vi "Simplified WB Spectrum Sense (Averaged).vi"(7 "Averaging Parameters":T1={"averaging mode"=enum."RMS averaging", "weighting mode"=enum."Linear", "number of averages"=10} {"number of averages" min=1}, 9 "Display Settings":cluster{"display unit":u16, "log/linear":u16}={"display unit"=2, "log/linear"=2} {"log/linear" items=["Linear", "dB", "dBm"]; "display unit" items=["Vrms", "Vpk", "Vrms^2", "Vpk^2", "Vrms/rtHz", "Vpk/rtHz", "Vrms^2/Hz", "Vpk^2/Hz"]}, 10 "Rx Parameters":T2={"IQ Sampling\nRate [S/sec]"=1000000.0, "Acq Duration [sec]"=0.001, "Start Carrier [Hz]"=88000000.0, "Stop Carrier [Hz]"=108000000.0, "Gain [dB]"=25.0, "Active Antenna"="RX2", "Reference Source"="Internal", "Timebase Source"="Internal"} {"Gain [dB]" format="%#_4g"; "Stop Carrier [Hz]" min=50000000.0 max=6000000000.0 step=1000.0 format="%#.15p"; "Start Carrier [Hz]" min=50000000.0 max=6000000000.0 step=1000.0 format="%#.15p"; "Acq Duration [sec]" min=0.0 step=0.001 format="%#.6p"; "IQ Sampling\nRate [S/sec]" format="%#_6p"}, 11 "USRP IP Address":refnum<k15>="192.168.12.4") -> (0 "error out":errorcluster, 2 "FFT Power Spectrum":cluster{"f0":dbl, "df":dbl, "IQ":dbl[]}(graph)={"f0"=87750000.0, "df"=1000.0, "IQ"=array[20500 elements]})   [LabVIEW 2011]
panel:
  in  "stop":bool
  # "Wideband Spectrum (Averaged)"
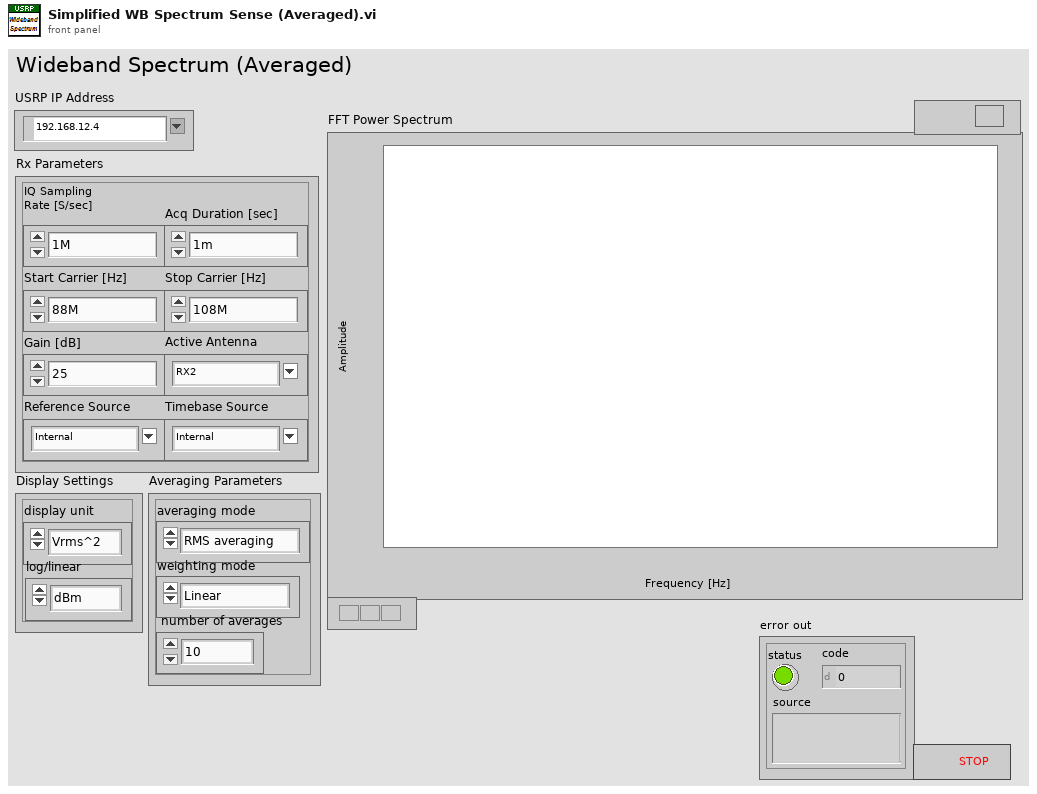
[diagram p1: front panel]
types:
  T1 = cluster{"averaging mode":enum16{"No averaging", "Vector averaging", "RMS averaging", "Peak hold"}, "weighting mode":enum16{"Linear", "Exponential"}, "number of averages":u32}
  T2 = cluster{"IQ Sampling\nRate [S/sec]":dbl, "Acq Duration [sec]":dbl, "Start Carrier [Hz]":dbl, "Stop Carrier [Hz]":dbl, "Gain [dB]":dbl, "Active Antenna":string, "Reference Source":string, "Timebase Source":string}
  T3 = typedef "subFrameParams.ctl" = cluster{"IQ Rate":dbl, "Frames":i32, "Length of Subset":i32, "Start Index of Subset":i32, "Start Carrier [Hz]":dbl, "Stop Carrier [Hz]":dbl, "Acq Duration [sec]":dbl}
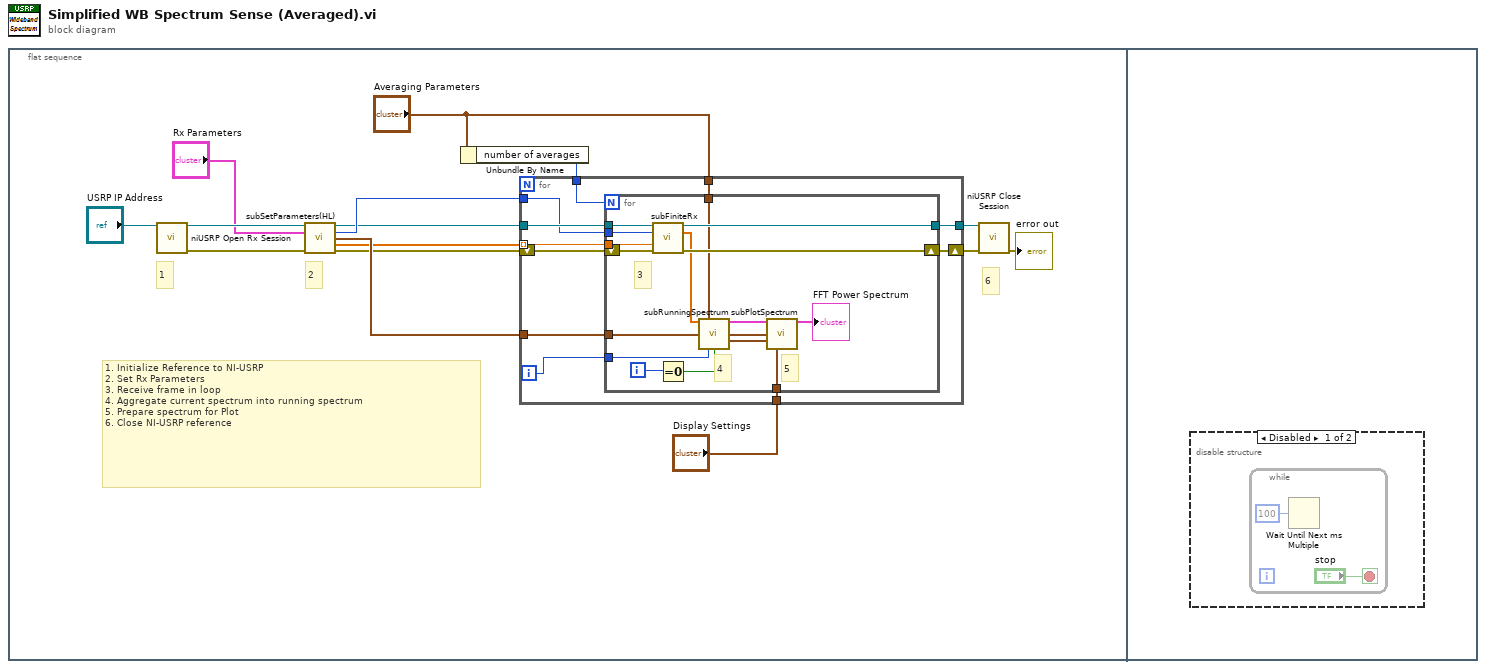
[diagram p0: block diagram]
diagram:
  n1 = flat-sequence {
    frame #0 {
      # "6"
      # "2"
      # "1"
      # "1. Initialize Reference to NI-USRP\n2. Set Rx Parameters\n3. Receive frame in loop\n4. Aggregate current spectrum into running spectrum\n5. Prepare spectrum for Plot\n6. Close NI-USRP reference"
      n2 = call <instrlib>:"niUSRP Open Rx Session.vi"("device names"="USRP IP Address") -> ("session handle out"=w10:refnum<k15>, "error out"=w9:errorcluster)  [unwired: 13 in]
      n3 = call "subSetParameters(HL).vi"("IVI Refnum in"=w10, "Rx Parameters"="Rx Parameters", "error in (no error)"=w9) -> ("IVI Refnum out"=w2:refnum<k15>, "samples per acquisition"=w12:i32, "Frame Parameters"=w7:T3, "test carrier frequencies"=w6:dbl[], "error out"=w1:errorcluster)  [unwired: 8 in]
      n4 = Unbundle By Name("Averaging Parameters") -> ("number of averages"=w4:u32)
      n5 = for {
        tunnel: w2 -> [w26]
        tunnel: w12 -> [w20]
        tunnel: [w25] -> w14
        shift-right: [w19] -> w13
        shift-left: w1 -> [w24]
        tunnel: w7 -> [w23]
        tunnel: w6 -> [w22] mode=indexing
        tunnel: "Display Settings" -> [w21]
        tunnel: w4 -> [w18]
        tunnel: "Averaging Parameters" -> [w17]
        i -> [w16]
        n6 = for {
          N: w18 -> [_]
          tunnel: w26 -> [w43]
          tunnel: [w42] -> w25
          tunnel: w16 -> [w41]
          tunnel: w23 -> [w37]
          tunnel: w22 -> [w36]
          tunnel: w21 -> [w33]
          tunnel: w20 -> [w32]
          shift-right: [w31] -> w19
          shift-left: w24 -> [w40]
          tunnel: w17 -> [w30]
          i -> [w28]
          # "5"
          # "4"
          # "3"
          n7 = call "subFiniteRx.vi"("IVI Refnum in"=w43, "Number of Samples"=w32, "Carrier Frequency"=w36, "error in (no error)"=w40) -> ("IVI Refnum out"=w42:refnum<k15>, "data"=w27:cdb[], "error out"=w31:errorcluster)  [unwired: 9 in]
          n8 = Equal To 0?(x=w28) -> (x = 0?=w29:bool)
          n9 = call "subRunningSpectrum.vi"("Input Baseband IQ"=w27, "averaging parameters"=w30, "restart averaging"=w29, "Frame Parameters"=w37, "Iteration"=w41) -> ("Spectrum to Plot"=w39:cluster{"f0":dbl, "df":dbl, "IQ":dbl[]}, "Frame Parameters out"=w35:T3, "window properties"=w34:cluster{"eq noise BW":dbl, "coherent gain":dbl})  [unwired: 7 in, 1 out]
          n10 = call "subPlotSpectrum.vi"("Spectrum to Plot"=w39, "Frame Parameters"=w35, "window properties"=w34, "Display"=w33) -> ("Spectrum to Plot"=→"FFT Power Spectrum":cluster{"f0":dbl, "df":dbl, "IQ":dbl[]})  [unwired: 11 in]
        }
      }
      n11 = call <instrlib>:"niUSRP Close Session.vi"("session handle"=w14, "error in (no error)"=w13) -> ("error out"=→"error out":errorcluster)  [unwired: 13 in]
    }
    frame #1 {
      n12 = disable-structure shown="Disabled" {
        frame Disabled {
          n13 = while {
            stop <- "stop" stop-if-true
            n14 = Wait Until Next ms Multiple(millisecond multiple=u32 100) -> ()  [unwired: 1 out]
          }
        }
        frame Enabled {
        }
      }
    }
  }
